vi "User_Defined_Test_TargetMet.vi"() -> (3 "Unit Test Framework Results":T1)   [LabVIEW 2016]
doc: "Use this template to create a user-defined test VI. Define your test requirements and wire the results to the <b>Result (Test)</b> control. Do not modify the <b>Unit Test Framework Results</b> indicator."
uses:
  <vilib>/utf/common/utf_test_result_troll.ctl
  <vilib>/utf/common/utf_test_result.ctl
  <vilib>/utf/common/utf_test_result_failure.ctl
  <vilib>/utf/common/utf_test_comparison_operators.ctl
  <vilib>/utf/common/utf_vi_tag.ctl
  <vilib>/Control Software Solutions Ltd/UTF Helper/SubVIs/UTF I32 Equals.vi
  MyPAM Controller/controllerLibrary.lvlib
  <vilib>/Control Software Solutions Ltd/UTF Helper/Unit Test Helper.lvlib
  <vilib>/utf/NI_UnitTestFramework.lvlib
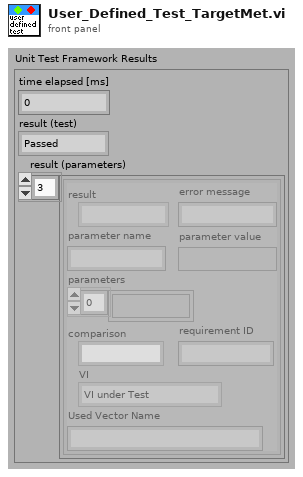
[diagram p1: front panel]
types:
  T1 = typedef "NI_UnitTestFramework.lvlib/utf_test_result_troll.ctl" = cluster{"time elapsed [ms]":u32, "result (test)":T2, "result (parameters)":T3[]}
  T2 = typedef "NI_UnitTestFramework.lvlib/utf_test_result.ctl" = enum16{"Passed", "Failed", "Error", "Skipped", "Not Processed"}
  T3 = typedef "NI_UnitTestFramework.lvlib/utf_test_result_failure.ctl" = cluster{"result":T2, "error message":string, "parameter name":string, "parameter value":variant, "parameters":variant[], "comparison":T4, "requirement ID":string, "VI":T5, "Used Vector Name":string}
  T4 = typedef "NI_UnitTestFramework.lvlib/utf_test_comparison_operators.ctl" = enum16{"=", "!=", ">", ">=", "<", "<=", "range", "symmetric tolerance", "asymmetric tolerance", "string contains", "string not contain", "array size", "string length", "array range", "by element", "array range (limit array)", "user-defined", "array contains", "array not contain", "vector length", "= (elm)", "!= (elm)", "= (case insensitive)", "!= (case insensitive)"}
  T5 = typedef "NI_UnitTestFramework.lvlib/utf_vi_tag.ctl" = enum16{"Setup VI", "VI under Test", "Teardown VI"}
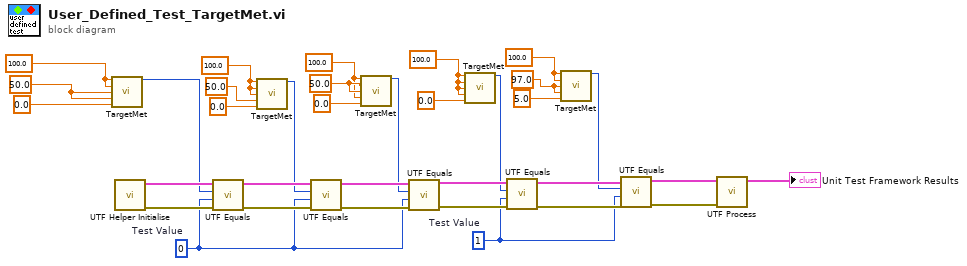
[diagram p0: block diagram]
diagram:
  w3 = 97.0 ("Target x (mm)")
  w11 = 100.0 ("Target x (mm)")
  w4 = 1  # Test Value
  w12 = 100.0 ("Target x (mm)")
  w2 = 50.0 ("Target x (mm)")
  w1 = 100.0 ("Target x (mm)")
  w19 = 100.0 ("Target x (mm)")
  w15 = 0  # Test Value
  w23 = 50.0 ("Target x (mm)")
  w24 = 100.0 ("Target x (mm)")
  n1 = call "TargetMet.vi"("Target x (mm)"=w24, "Target y (mm)"=w24, "Current x (mm)"=w23, "Current y (mm)"=w23, "Dead Zone (mm)"=0.0) -> ("out"=w22:i32)  [unwired: 10 in]
  n2 = call <vilib>:"UTF Helper Initialise.vi"() -> ("error out"=w32:errorcluster, "results array"=w33:T3[])  [unwired: 10 in]
  n3 = call-poly <vilib>:"UTF Equals.vi"("error in (no error)"=w32, "Test Value"=w15, "Input"=w22, "Input Results"=w33) -> ("error out"=w30:errorcluster, "Output Results"=w31:T3[])  [unwired: 6 in]
  n4 = call "TargetMet.vi"("Target x (mm)"=w19, "Target y (mm)"=w19, "Current x (mm)"=w19, "Current y (mm)"=50.0 ("Target x (mm)"), "Dead Zone (mm)"=0.0) -> ("out"=w18:i32)  [unwired: 10 in]
  n5 = call-poly <vilib>:"UTF Equals.vi"("error in (no error)"=w30, "Test Value"=w15, "Input"=w18, "Input Results"=w31) -> ("error out"=w28:errorcluster, "Output Results"=w29:T3[])  [unwired: 6 in]
  n6 = call "TargetMet.vi"("Target x (mm)"=w1, "Target y (mm)"=w2, "Current x (mm)"=w2, "Current y (mm)"=w1, "Dead Zone (mm)"=0.0) -> ("out"=w16:i32)  [unwired: 10 in]
  n7 = call-poly <vilib>:"UTF Equals.vi"("error in (no error)"=w28, "Test Value"=w15, "Input"=w16, "Input Results"=w29) -> ("error out"=w26:errorcluster, "Output Results"=w27:T3[])  [unwired: 6 in]
  n8 = call "TargetMet.vi"("Target x (mm)"=w12, "Target y (mm)"=w12, "Current x (mm)"=w12, "Current y (mm)"=w12, "Dead Zone (mm)"=0.0) -> ("out"=w13:i32)  [unwired: 10 in]
  n9 = call-poly <vilib>:"UTF Equals.vi"("error in (no error)"=w26, "Test Value"=w4, "Input"=w13, "Input Results"=w27) -> ("error out"=w6:errorcluster, "Output Results"=w9:T3[])  [unwired: 6 in]
  n10 = call "TargetMet.vi"("Target x (mm)"=w11, "Target y (mm)"=w11, "Current x (mm)"=w3, "Current y (mm)"=w3, "Dead Zone (mm)"=5.0) -> ("out"=w5:i32)  [unwired: 10 in]
  n11 = call-poly <vilib>:"UTF Equals.vi"("error in (no error)"=w6, "Test Value"=w4, "Input"=w5, "Input Results"=w9) -> ("error out"=w7:errorcluster, "Output Results"=w8:T3[])  [unwired: 6 in]
  n12 = call <vilib>:"UTF Process.vi"("error in (no error)"=w7, "results array"=w8) -> ("Unit Test Framework Results"=→"Unit Test Framework Results":T1)  [unwired: 9 in]
